vi "ToString.vi"(8 "error in (no error)":errorcluster, 11 "IsTrue in":refnum<class "IsTrue.lvclass">) -> (0 "error out":errorcluster, 2 "String":string, 3 "IsTrue out":refnum<class "IsTrue.lvclass">)   [LabVIEW 2017, in "Transparent Assertions.lvlib" / "Constraints.lvlib" / "IsTrue.lvclass"]
doc: "Returns a string representation of the object."
uses:
  IsTrue.lvclass
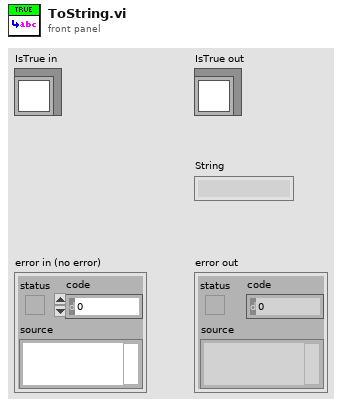
[diagram p1: front panel]
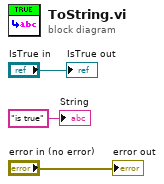
[diagram p0: block diagram]
diagram:
  "error out" <- "error in (no error)"
  "IsTrue out" <- "IsTrue in"
  "String" <- "is true" ("String")
